vi "create_wf.vi"() -> ()   [LabVIEW 2013]
uses:
  wf_tools/stage.ctl
  <vilib>/Utility/xml.llb/Write to XML File(string).vi
  wf_tools/wf_tools.lvlib
panel:
  in  "Save":bool
  out "init":bool
  in  "Build":bool
  in  "Stop Button":bool
  in  "Tab Control":T1(tab)=enum."electrodes"
  out "num_electrodes":i32=15
  in  "cell length":dbl=0.05 caption="cell length (m)" format="%#_6p"
  in  "input":T2(array[cluster])=[{"final vel. (m/s)"=0.0, "distance (m)"=0.1, "hold (s)"=1e-05}, {"final vel. (m/s)"=1000.0, "distance (m)"=0.025, "hold (s)"=0.0}] {"hold (s)" format="%#_6p"; "distance (m)" format="%#_6p"; "final vel. (m/s)" format="%#_6p"}
  in  "initial velocity":dbl=2000.0 caption="initial velocity (m/s)" format="%#_6p"
  in  "dt":dbl=2.5e-08 caption="dt (s)" format="%#_6p"
  in  "electrodes/ cell":i32=6
  out "num_steps":i32=6400
  out "xt":cluster{"time":dbl[], "velocity":dbl[]}[](graph)
  out "valid":bool=TRUE
  out "total d":dbl=0.125 caption="final position (m)" format="%#_6p"
  out "total t":dbl=0.00016 caption="total time (s)" format="%#_6p"
  out "max a":dbl=20000000.0 caption="max accel. (m /s^2)"
  out "stages":T3[](array[typedef])=[{"v_i (m/s)"=2000.0, "v_f (m/s)"=0.0, "a (m / s^2)"=-20000000.0, "d (m)"=0.1, "t (s)"=0.0001}, {"v_i (m/s)"=0.0, "v_f (m/s)"=0.0, "a (m / s^2)"=0.0, "d (m)"=0.0, "t (s)"=1e-05}, {"v_i (m/s)"=0.0, "v_f (m/s)"=1000.0, "a (m / s^2)"=20000000.0, "d (m)"=0.025, "t (s)"=5e-05}] {"t (s)" format="%#_6e"; "v_i (m/s)" format="%#_6e"; "a (m / s^2)" format="%#_6e"; "d (m)" format="%#_6e"; "v_f (m/s)" format="%#_6e"}
  in  "ramp tail (s)":dbl format="%#_6p"
  out "el":waveform(dbl)[](graph)=[{"t0"=timestamp(0 s since 1904-01-01), "dt"=2.5e-08, "Y"=array[6400 elements]}, {"t0"=timestamp(0 s since 1904-01-01), "dt"=2.5e-08, "Y"=array[6400 elements]}, {"t0"=timestamp(0 s since 1904-01-01), "dt"=2.5e-08, "Y"=array[6400 elements]}, {"t0"=timestamp(0 s since 1904-01-01), "dt"=2.5e-08, "Y"=array[6400 elements]}, {"t0"=timestamp(0 s since 1904-01-01), "dt"=2.5e-08, "Y"=array[6400 elements]}, {"t0"=timestamp(0 s since 1904-01-01), "dt"=2.5e-08, "Y"=array[6400 elements]}]
  out "el freq":waveform(dbl)(graph)={"t0"=timestamp(0 s since 1904-01-01), "dt"=2.5e-08, "Y"=array[6400 elements]}
  in  "ramp head (s)":dbl=1e-05 format="%#_6p"
  in  "phase_c":dbl=-0.5 caption="phase (/ 2 pi)"
  out "corr freq":waveform(dbl)(graph)={"t0"=timestamp(0 s since 1904-01-01), "dt"=2.5e-08, "Y"=array[6400 elements]}
  out "corr":waveform(dbl)[](graph)=[{"t0"=timestamp(0 s since 1904-01-01), "dt"=2.5e-08, "Y"=array[6400 elements]}]
  in  "add func":bool
  in  "f(x, t)":string="-5 * exp(\n-(x-4E-2)^2/\n(2 * (2E-3^2)))"
  # "Rydberg Stark decelerator"
  # "Use the 'input' tab to specify the electrode configuration and desired acceleration/ deceleration stages.   The electrodes are equally spaced and grouped into cells of 'n' electrodes, where every i'th electrode is connected to the (i + n)'th. \n\nAfter making changes to the input settings ensure that the 'valid' indicator is lit then press 'Build' to solve the equations of motion for each stage (output to the 'sequence' tab) and to find the position of the trap centre as a function of time.\n\nThe trap position is translated into its phase with respect to the position of each electrode, which in turn gives the electrode waveforms (these are displayed on the 'electrodes' tab).  The waveforms can be linearly ramped on and off using the  'apply ramp' settings.\n\nThe 'correction' tab shows the waveform for the top electrode, which modulates to correct for a weakening of the trap as it passes over the regions between electrodes.  The frequency of the correction waveform is n times larger than that for the electrodes.  An arbitrary function that varies with either or both the trap position (x) and time (t) can be added to this. \n\nTo view the changes, press 'Build' after modifying the input, ramp, add function, amplitudes, and offset settings. \n\nWaveforms scaled to between +/- 1.  Set amplitude and offset with hardware.\n\nSave as a *.wf file (XML).\n\nNB.  The functions of this vi are available for use as a subVI in wf_tools:create.vi"
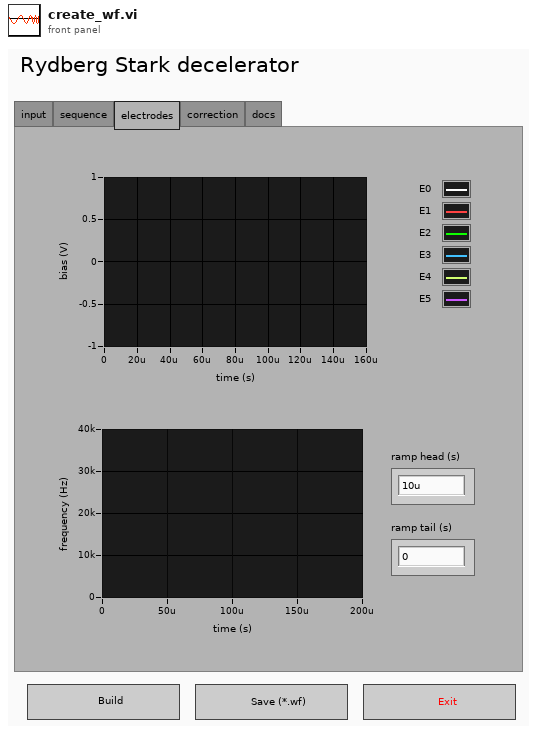
[diagram p1: front panel]
types:
  T1 = enum32{"input", "sequence", "electrodes", "correction", "docs"}
  T2 = cluster{"final vel. (m/s)":dbl, "distance (m)":dbl, "hold (s)":dbl}[]
  T3 = typedef "wf_tools.lvlib/stage.ctl" = cluster{"v_i (m/s)":dbl, "v_f (m/s)":dbl, "a (m / s^2)":dbl, "d (m)":dbl, "t (s)":dbl}
  T4 = enum8{"Enabled", "Disabled", "Disabled and Grayed Out"}
  T5 = cluster{"time":dbl[], "position":dbl[], "velocity":dbl[]}
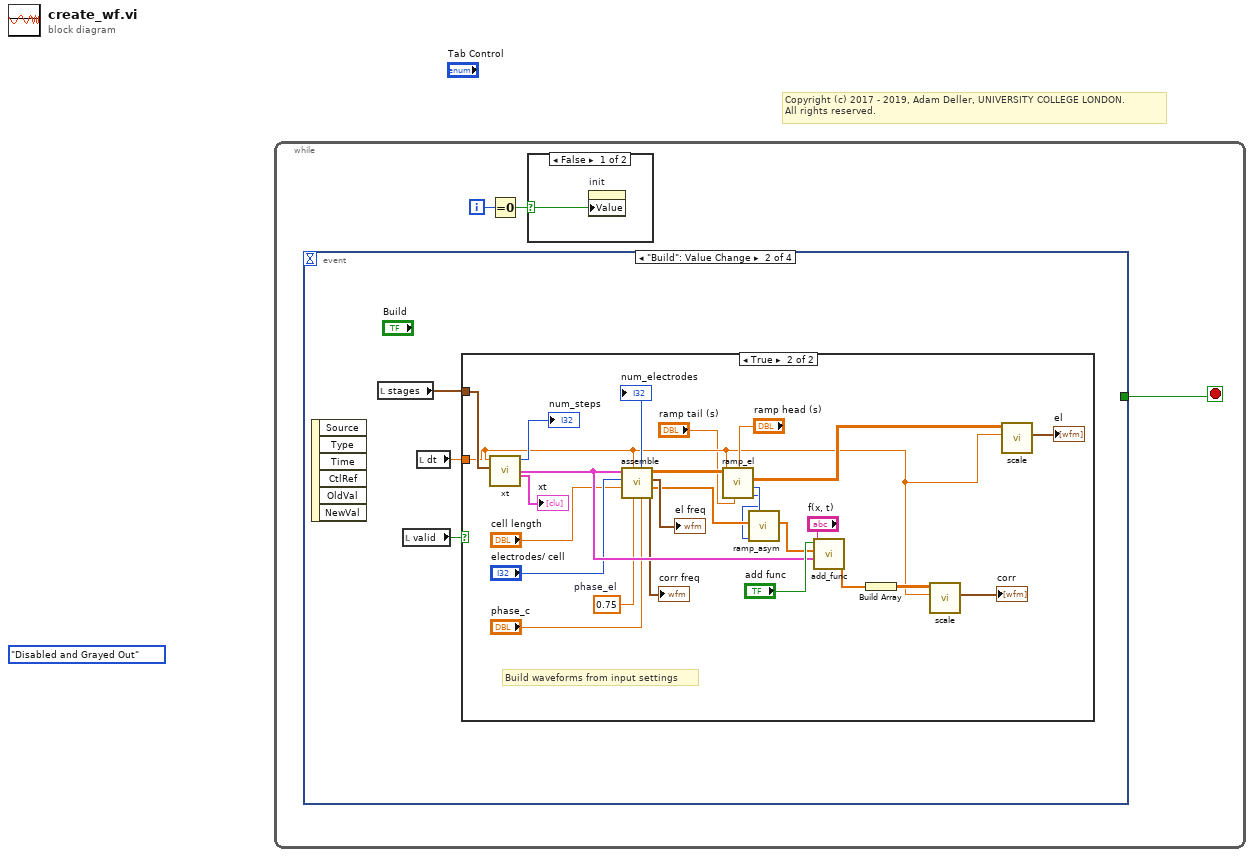
[diagram p0: block diagram]
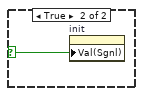
[diagram p2: hidden frame]
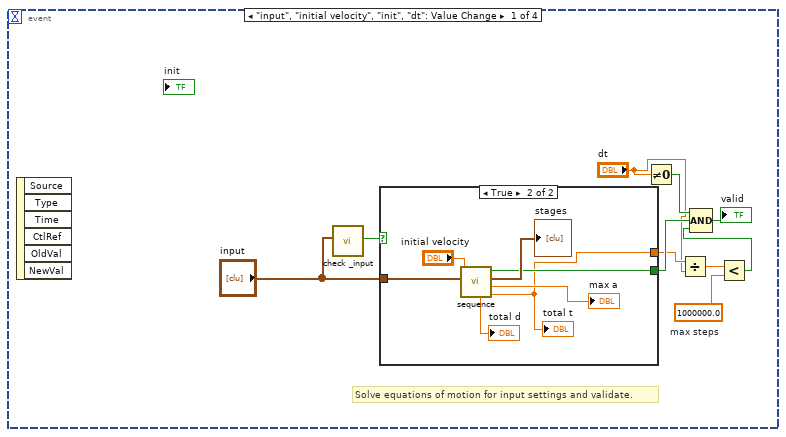
[diagram p3: hidden frame]
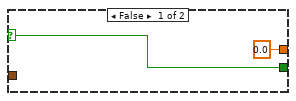
[diagram p4: hidden frame]
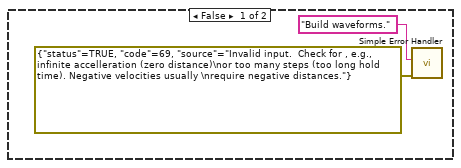
[diagram p5: hidden frame]
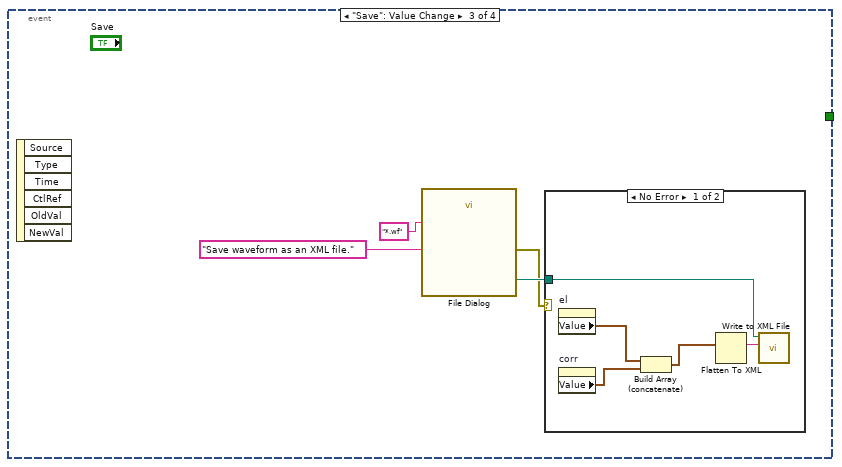
[diagram p6: hidden frame]
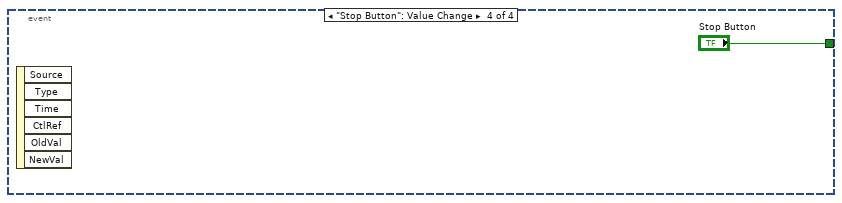
[diagram p8: hidden frame]
diagram:
  (unwired) T4."Disabled and Grayed Out" ("Disabled")
  # "Copyright (c) 2017 - 2019, Adam Deller, UNIVERSITY COLLEGE LONDON.\nAll rights reserved."
  n1 = while {
    i -> [w2]
    stop <- w3 stop-if-true
    n2 = event shown="[1] \"Build\": Value Change" {
      selector: _ -> [_ _ _ _]
      dyn-events: _ -> [_ _ _ _]
      timeout: _ -> [_ _ _ _]
      tunnel: [_ _ _ "Stop Button"] -> w3
      event "input", "initial velocity", "init", "dt": Value Change {
        w7 = 1000000.0  # max steps
        # "Solve equations of motion for input settings and validate."
        n3 = event-data() -> ()  [unwired: 1 in, 6 out]
        n4 = call "check _input.vi"("input"="input") -> ("valid"=w14:bool)  [unwired: 10 in]
        n5 = case shown="True" w14 {
          selector: w14 -> [w17 _]
          tunnel: "input" -> [_ w24]
          tunnel: [w17 w21] -> w11
          tunnel: [0.0 ("total t") w18] -> w10
          frame False {
          }
          frame True {
            n6 = call "sequence.vi"("input"=w24, "initial vel."="initial velocity") -> ("total t"=w18:dbl, "max a"=→"max a":dbl, "stages"=→"stages":T3[], "valid"=w21:bool, "total d"=→"total d":dbl)  [unwired: 5 in]
            "total t" <- w18
          }
        }
        n7 = Not Equal To 0?(x="dt") -> (x != 0?=w12:bool)
        n8 = Divide(x=w10, y="dt") -> (x/y=w8:dbl)
        n9 = Less?(x=w8, y=w7) -> (x < y?=w6:bool)
        n10 = Compound Arithmetic op=AND(w12, w11, w6) -> (→"valid":bool)
      }
      event "Build": Value Change {
        n11 = event-data() -> ()  [unwired: 1 in, 6 out]
        n12 = local read "stages"() -> (w26:T3[])
        n13 = local read "valid"() -> (w27:bool)
        n14 = local read "dt"() -> (w25:dbl)
        n15 = case shown="True" w27 {
          tunnel: w26 -> [_ w51]
          tunnel: w25 -> [_ w35]
          frame False {
            n16 = call <vilib>:"Simple Error Handler.vi"("error source (\" \")"="Build waveforms." ("error source (\" \")"), "error in (no error)"=errorcluster {"status"=TRUE, "code"=69, "source"="Invalid input.  Check for , e.g., infinite accelleration (zero distance)\nor too many steps (too long hold time). Negative velocities usually \nrequire negative distances."}) -> ()  [unwired: 3 in, 5 out]
          }
          frame True {
            w40 = 0.75  # phase_el
            # "Build waveforms from input settings"
            n17 = call "xt.vi"("stages"=w51, "dt (s)"=w35) -> ("XT"=→"xt":cluster{"time":dbl[], "velocity":dbl[]}[], "output"=w46:T5, "num_steps"=→"num_steps":i32)  [unwired: 7 in]
            n18 = call "assemble.vi"("corr phase"="phase_c", "el phase"=w40, "dt"=w35, "cell length"="cell length", "electrodes/ cell"="electrodes/ cell", "input"=w46) -> ("corr freq"=→"corr freq":waveform(dbl), "correction"=w33:dbl[], "el freq"=→"el freq":waveform(dbl), "electrodes"=w38:dbl[][], "num_electrodes"=→"num_electrodes":i32)  [unwired: 1 in]
            n19 = call "ramp_el.vi"("ramp tail (s)"="ramp tail (s)", "dt"=w35, "ramp head (s)"="ramp head (s)", "wf_in"=w38) -> ("num_tail"=w30:i32, "num_head"=w34:i32, "wf_out"=w37:dbl[][])  [unwired: 5 in]
            n20 = call "ramp_asym.vi"("num_tail"=w30, "num_head"=w34, "wf_in"=w33) -> ("wf_out"=w32:dbl[])  [unwired: 8 in]
            n21 = call "add_func.vi"("f(x, t)"="f(x, t)", "output"=w46, "wf_in"=w32, "apply"="add func") -> ("wf_out"=w48:dbl[])  [unwired: 6 in, 1 out]
            n22 = Build Array(w48) -> (w54:dbl[][])
            n23 = call "scale.vi"("dt"=w35, "waveforms"=w54) -> ("el"=→"corr":waveform(dbl)[])  [unwired: 9 in]
            n24 = call "scale.vi"("dt"=w35, "waveforms"=w37) -> ("el"=→"el":waveform(dbl)[])  [unwired: 9 in]
          }
        }
      }
      event "Save": Value Change {
        n25 = event-data() -> ()  [unwired: 1 in, 6 out]
        n26 = call "File Dialog"("prompt"="Save waveform as an XML file.", "pattern (all files)"="*.wf" ("pattern label")) -> ("selected path"=w59:path, "error out"=w56:errorcluster)  [unwired: 10 in, 2 out]
        n27 = case shown="No Error" w56 {
          tunnel: w59 -> [w63 _]
          frame No Error {
            n28 = property on="el" class="WFGraph (strict)"() -> ("Value"=w62:waveform(dbl)[])  [unwired: 2 in, 2 out]
            n29 = property on="corr" class="WFGraph (strict)"() -> ("Value"=w61:waveform(dbl)[])  [unwired: 2 in, 2 out]
            n30 = Build Array (concatenate)(w62, w61) -> (w60:waveform(dbl)[])
            n31 = Flatten To XML(anything=w60) -> (xml string=w64:string)
            n32 = call-poly <vilib>:"Write to XML File.vi"("XML Input"=w64, "XML File Path"=w63) -> ()  [unwired: 7 in, 3 out]
          }
          frame Error {
          }
        }
      }
      event "Stop Button": Value Change {
        n33 = event-data() -> ()  [unwired: 1 in, 6 out]
      }
    }
    n34 = Equal To 0?(x=w2) -> (x = 0?=w1:bool)
    n35 = case shown="False" w1 {
      selector: w1 -> [w4 w5]
      frame False {
        n36 = property on="init" class="Bool (strict)"("Value"=w4) -> ()  [unwired: 2 in, 2 out]
      }
      frame True {
        n37 = property on="init" class="Bool (strict)"("Val(Sgnl)"=w5) -> ()  [unwired: 2 in, 2 out]
      }
    }
  }
